vi "Initialize.vi"(8 "error in (no error)":errorcluster, 9 "Reset (True)":bool=TRUE, 10 "ID Query (True)":bool=TRUE, 11 "VISA resource name":refnum<visa-resource-name>) -> (0 "error out":errorcluster, 3 "VISA resource name out":refnum<visa-resource-name>)   [LabVIEW 2015, in "SDG X Series.lvlib"]
doc: "Establishes communication with the instrument and optionally performs an instrument identification query and/or an instrument reset. It also places the instrument in a default state needed for other instrument driver operations. Therefore, call this VI before calling other instrument driver VIs for this instrument. Generally, you need to call the Initialize VI only once at the beginning of an application."
uses:
  <instrlib>/SDG X Series/SDG X Series.lvlib
panel:
  # "(c) 2017 SIGLENT TECHNOLOGIES CO.,LTD. ALL RIGHTS RESERVED."
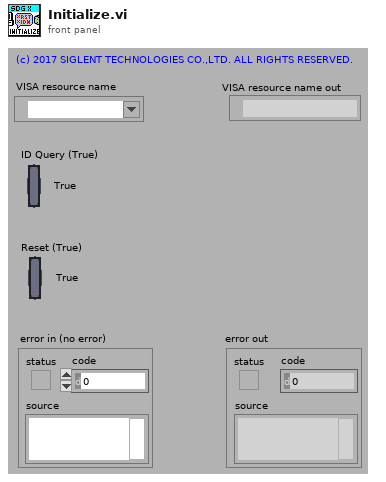
[diagram p1: front panel]
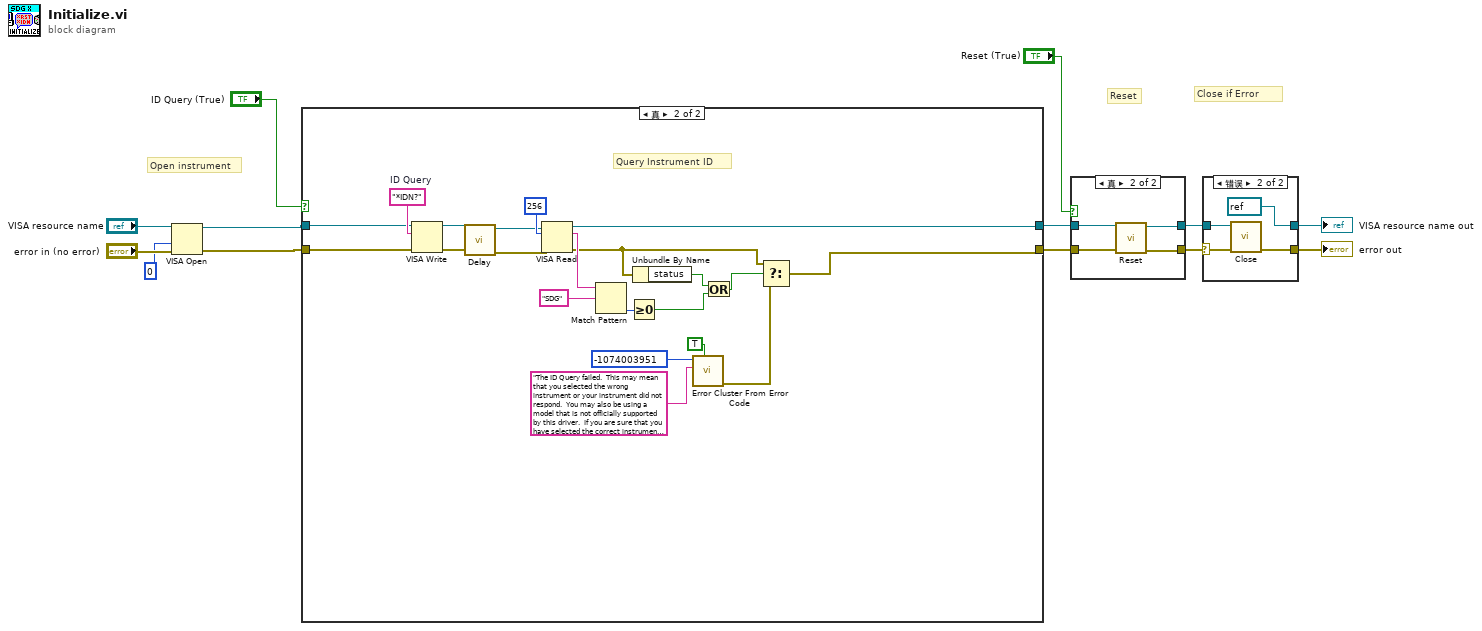
[diagram p0: block diagram]
diagram:
  # "Reset"
  # "Close if Error"
  # "Open instrument"
  n1 = VISA Open(access mode=u32 0, error in (no error)="error in (no error)", VISA resource name="VISA resource name") -> (VISA resource name=w3:refnum<visa-resource-name>, error out=w2:errorcluster)  [unwired: 2 in]
  n2 = case shown="真" "ID Query (True)" {
    tunnel: [w14 w21] -> w8
    tunnel: [w15 w20] -> w9
    tunnel: w3 -> [w15 w23]
    tunnel: w2 -> [w14 w22]
    frame False {
    }
    frame True {
      w34 = "*IDN?"  # ID Query
      # "Query Instrument ID"
      n3 = VISA Write(VISA resource name=w23, write buffer=w34, error in (no error)=w22) -> (VISA resource name out=w18:refnum<visa-resource-name>, error out=w19:errorcluster)  [unwired: 1 out]
      n4 = call <instrlib>:"Delay.vi"("error in (no error)"=w19, "VISA resource name"=w18) -> ("error out"=w16:errorcluster, "VISA resource name out"=w17:refnum<visa-resource-name>)  [unwired: 8 in]
      n5 = VISA Read(VISA resource name=w17, byte count=u32 256, error in (no error)=w16) -> (VISA resource name out=w20:refnum<visa-resource-name>, read buffer=w25:string, error out=w24:errorcluster)  [unwired: 1 out]
      n6 = Match Pattern(string=w25, regular expression="SDG") -> (offset past match=w29:i32)  [unwired: 1 in, 3 out]
      n7 = Greater Or Equal To 0?(x=w29) -> (x >= 0?=w27:bool)
      n8 = Unbundle By Name(w24) -> ("status"=w28:bool)
      n9 = call <vilib>:"Error Cluster From Error Code.vi"("show call chain? (False)"=TRUE, "error message (\"\")"="The ID Query failed.  This may mean that you selected the wrong instrument or your instrument did not respond.  You may also be using a model that is not officially supported by this driver.  If you are sure that you have selected the correct instrument and it is responding, try disabling the ID Query." ("Source (VI Name)"), "error code (0)"=-1074003951 ("Code")) -> ("error out"=w33:errorcluster)  [unwired: 6 in]
      n10 = Or(x=w28, y=w27) -> (x .or. y?=w26:bool)
      n11 = Select(t=w24, s=w26, f=w33) -> (s? t:f=w21:errorcluster)
    }
  }
  n12 = case shown="真" "Reset (True)" {
    tunnel: w8 -> [w37 w41]
    tunnel: [w37 w40] -> w7
    tunnel: w9 -> [w38 w42]
    tunnel: [w38 w39] -> w6
    frame False {
    }
    frame True {
      n13 = call <instrlib>:"Reset.vi"("error in (no error)"=w41, "VISA resource name"=w42) -> ("error out"=w40:errorcluster, "VISA resource name out"=w39:refnum<visa-resource-name>)  [unwired: 8 in]
    }
  }
  n14 = case shown="错误" w7 {
    selector: w7 -> [w43 w46]
    tunnel: w6 -> [w44 w47]
    tunnel: [w44 refnum<visa-resource-name> refnum ("VISA resource name out")] -> w11
    tunnel: [w43 w48] -> w10
    frame No Error {
    }
    frame Error {
      n15 = call <instrlib>:"Close.vi"("error in (no error)"=w46, "VISA resource name"=w47) -> ("error out"=w48:errorcluster)  [unwired: 9 in]
    }
  }
  "VISA resource name out" <- w11
  "error out" <- w10
